vi "Resolve Imports.vi"(4 "Include Paths":path[](array[path]), 6 "Source .proto":path, 7 "Enumerations in":map{string, T1}(c390), 8 "error in (no error)":errorcluster, 9 "Messages in":map{string, T5}(c390), 10 "Segments in":T3[](array[typedef]), 11 "ProtoParser in":refnum<class "ProtoParser.lvclass">) -> (0 "error out":errorcluster, 1 "Messages":map{string, T5}(c390), 2 "Segments":T3[](array[typedef]), 3 "ProtoParser out":refnum<class "ProtoParser.lvclass">, 5 "Enumerations":map{string, T1}(c390))   [LabVIEW 2020, in "LV-Protoc.lvlib" / "ProtoParser.lvclass"]
uses:
  ProtoParser.lvclass
  Segment Type.ctl
  LV-Protoc.lvlib
  Raw Segment.ctl
  LV-Proto/Proto Type.ctl
  LV-Proto/LV-Proto.lvlib
  LV-Proto/Field.ctl
  LV-Proto/Message.ctl
  LV-Proto/Enum Value.ctl
  LV-Proto/Enumeration.ctl
  LV-Proto/Type.ctl
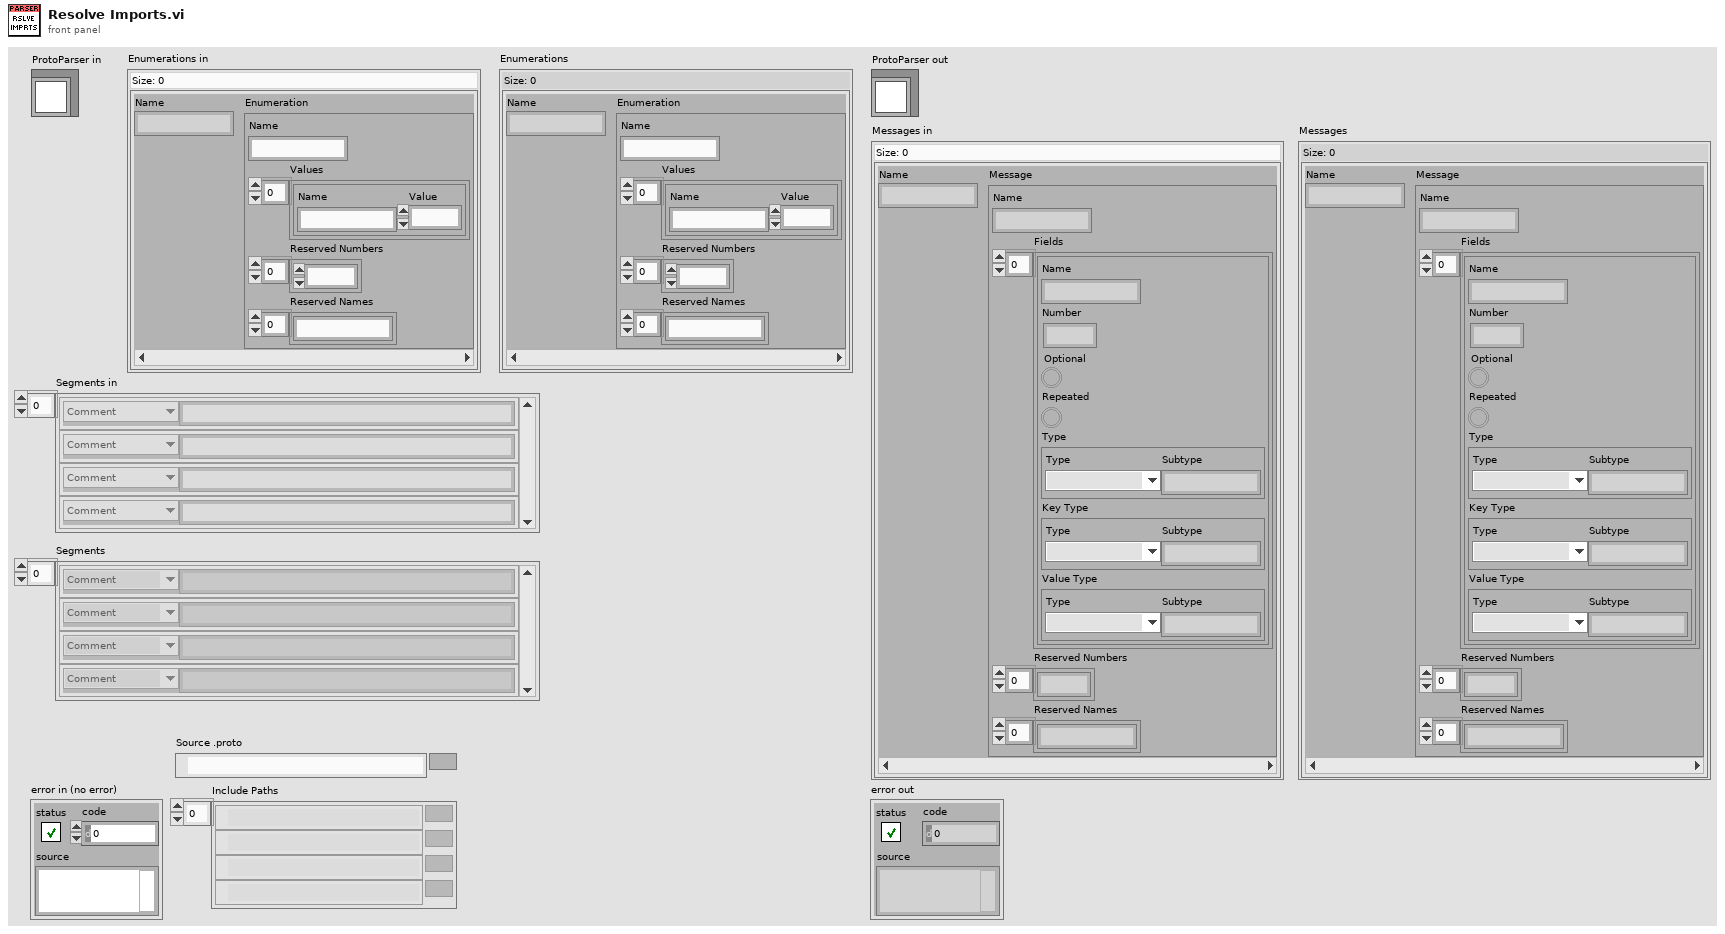
[diagram p1: front panel]
types:
  T1 = typedef "LV-Proto.lvlib/Enumeration.ctl" = cluster{"Name":string, "Values":T2[], "Reserved Numbers":u32[], "Reserved Names":string[]}
  T2 = typedef "LV-Proto.lvlib/Enum Value.ctl" = cluster{"Name":string, "Value":i32}
  T3 = typedef "LV-Protoc.lvlib/Raw Segment.ctl" = cluster{"Type":T4, "Text":string}
  T4 = typedef "LV-Protoc.lvlib/Segment Type.ctl" = enum16{"Comment", "Message Open", "Enum Open", "Message Close", "Enum Close", "Field", "Syntax", "Import", "Enum Value", "Package", "Reserved"}
  T5 = typedef "LV-Proto.lvlib/Message.ctl" = cluster{"Name":string, "Fields":T6[], "Reserved Numbers":u32[], "Reserved Names":string[]}
  T6 = typedef "LV-Proto.lvlib/Field.ctl" = cluster{"Name":string, "Number":u32, "Optional":bool, "Repeated":bool, "Type":T7, "Key Type":T7, "Value Type":T7}
  T7 = typedef "LV-Proto.lvlib/Type.ctl" = cluster{"Type":T8, "Subtype":string}
  T8 = typedef "LV-Proto.lvlib/Proto Type.ctl" = enum16{"UNKNOWN", "double", "float", "int32", "int64", "uint32", "uint64", "sint32", "sint64", "fixed32", "fixed64", "sfixed32", "sfixed64", "bool", "string", "bytes", "enum", "map", "message"}
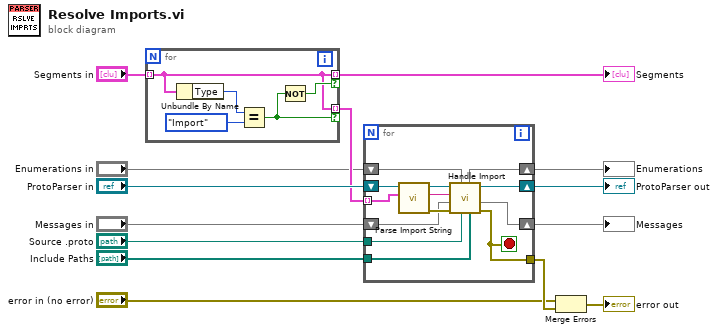
[diagram p0: block diagram]
diagram:
  n1 = for {
    tunnel: "Segments in" -> [w15] mode=indexing
    tunnel: [w15] -> w13 mode=indexing if=w16
    tunnel: [w15] -> w10 mode=indexing if=w17
    n2 = Unbundle By Name(w15) -> ("Type"=w19:T4)
    n3 = Equal?(x=w19, y=Segment_Type."Import") -> (x = y?=w17:bool)
    n4 = Not(x=w17) -> (.not. x?=w16:bool)
  }
  "Segments" <- w13
  n5 = for {
    shift-right: [w29] -> w11
    shift-left: "ProtoParser in" -> [w32]
    tunnel: w10 -> [w31] mode=indexing
    shift-right: [w23] -> w6
    shift-left: "Messages in" -> [w26]
    tunnel: "Include Paths" -> [w24]
    tunnel: "Source .proto" -> [w25]
    tunnel: [w22] -> w5
    shift-right: [w20] -> w1
    shift-left: "Enumerations in" -> [w21]
    stop <- w22 stop-if-true
    n6 = call "Parse Import String.vi"("Raw Segment"=w31, "ProtoParser in"=w32) -> ("error out"=w28:errorcluster, "Import String"=w27:string, "ProtoParser out"=w30:refnum<class "ProtoParser.lvclass">)  [unwired: 7 in]
    n7 = call "Handle Import.vi"("Search Paths"=w24, "Source .proto"=w25, "Enumerations in"=w21, "error in (no error)"=w28, "Messages in"=w26, "Import String"=w27, "ProtoParser in"=w30) -> ("error out"=w22:errorcluster, "Messages"=w23:map{string, T5}, "ProtoParser out"=w29:refnum<class "ProtoParser.lvclass">, "Enumerations"=w20:map{string, T1})  [unwired: 1 in]
  }
  "ProtoParser out" <- w11
  "Messages" <- w6
  "Enumerations" <- w1
  n8 = Merge Errors("error in (no error)", w5) -> (→"error out":errorcluster)
